vi "Apply Selected Labels to Control.vi"(8 "error in (no error)":errorcluster, 10 "Alternate Text Select (0)":i32, 11 "Cluster in":refnum<class "Cluster.lvclass">) -> (0 "error out":errorcluster, 3 "Cluster out":refnum<class "Cluster.lvclass">)   [LabVIEW 2017, in "Localization.lvlib" / "Cluster.lvclass"]
doc: "Use the information in the class to apply the selected alternate text from the Additional Labels to the control.\n\nChoose Movement Consulting, LLC"
uses:
  Cluster.lvclass
  C:/Apps/CMC/OpenSource/Localization/Control Info/Control Info.lvclass
  Control Info/Control Info.lvclass
  Localization.lvlib
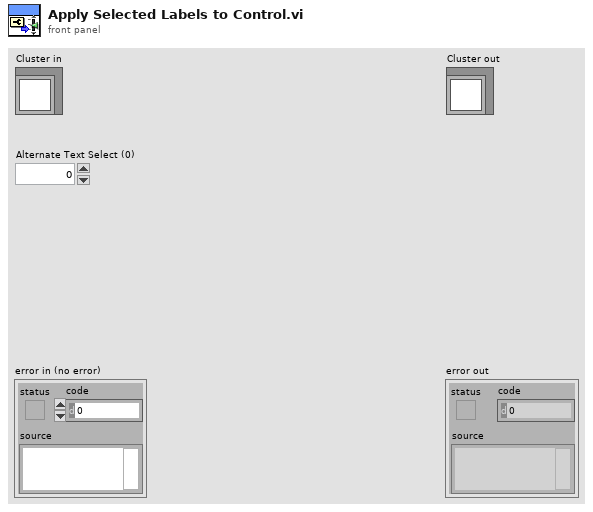
[diagram p1: front panel]
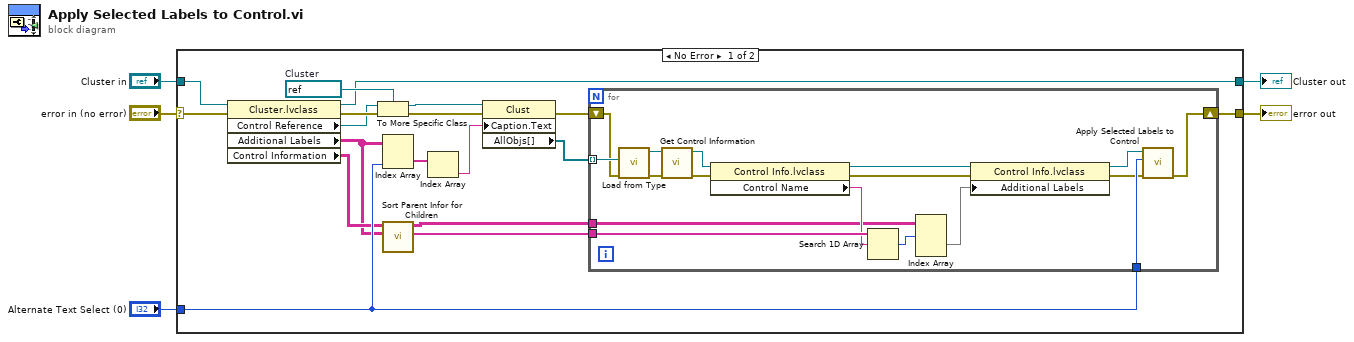
[diagram p0: block diagram]
diagram:
  n1 = case shown="No Error" "error in (no error)" {
    selector: "error in (no error)" -> [w18 w42]
    tunnel: "Cluster in" -> [w17 w41]
    tunnel: [w6 w42] -> w4
    tunnel: [w14 w41] -> w3
    tunnel: "Alternate Text Select (0)" -> [w12 _]
    frame No Error {
      w23 = refnum<vi> refnum  # Cluster
      n2 = property class="Cluster.lvclass"(reference=w17, error in=w18) -> (reference out=w14:refnum<class "Cluster.lvclass">, error out=w20:errorcluster, "Control Reference"=w19:refnum<vi>, "Additional Labels"=w10:string[][], "Control Information"=w11:string[][])
      n3 = To More Specific Class(target class=w23, reference=w19, error in=w20) -> (specific class reference=w22:refnum<vi>, error out=w21:errorcluster)
      n4 = Index Array(array=w10, index (col)=w12) -> (element=w15:string[])  [unwired: 1 in]
      n5 = call "Sort Parent Infor for Children.vi"("Additional Labels"=w10, "Control Information in"=w11) -> ("Control Names"=w9:string[], "Broken Out Additional Labels"=w8:string[][][])  [unwired: 7 in, 1 out]
      n6 = Index Array(array=w15) -> (element=w16:string)  [unwired: 1 in]
      n7 = property class="Clust"(reference=w22, error in=w21, "Caption.Text"=w16) -> (error out=w7:errorcluster, "AllObjs[]"=w13:refnum<vi>[])  [unwired: 1 out]
      n8 = for {
        tunnel: w13 -> [w40] mode=indexing
        tunnel: w12 -> [w39]
        tunnel: w9 -> [w36]
        tunnel: w8 -> [w34]
        shift-right: [w29] -> w6
        shift-left: w7 -> [w24]
        n9 = call "Load from Type.vi"("error in (no error)"=w24, "Control Reference"=w40) -> ("error out"=w27:errorcluster, "Control Info out"=w28:refnum<class "Control Info.lvclass">)  [unwired: 8 in]
        n10 = call-dynamic "Get Control Information.vi"("error in (no error)"=w27, "Control Info in"=w28) -> ("error out"=w26:errorcluster, "Control Info out"=w25:refnum<class "Control Info.lvclass">)  [unwired: 7 in, 1 out]
        n11 = property class="Control Info.lvclass"(reference=w25, error in=w26) -> (reference out=w37:refnum<class "Control Info.lvclass">, error out=w38:errorcluster, "Control Name"=w35:string)
        n12 = Search 1D Array(1D array=w36, element=w35) -> (index of element=w33:i32)  [unwired: 1 in]
        n13 = Index Array(array=w34, index (dim 0)=w33) -> (element=w32:string[][])  [unwired: 2 in]
        n14 = property class="Control Info.lvclass"(reference=w37, error in=w38, "Additional Labels"=w32) -> (reference out=w30:refnum<class "Control Info.lvclass">, error out=w31:errorcluster)
        n15 = call-dynamic "Apply Selected Labels to Control.vi"("error in (no error)"=w31, "Alternate Text Select (0)"=w39, "Control Info in"=w30) -> ("error out"=w29:errorcluster)  [unwired: 7 in, 1 out]
      }
    }
    frame Error {
    }
  }
  "error out" <- w4
  "Cluster out" <- w3
